vi "nodeInfo.get_process_info.vi"(5 "error in (no error)":errorcluster) -> (14 "numberProcs":i32, 15 "procNames":string[](array[string]), 16 "procID":i32[](array[numeric]), 17 "procMemory":i32[](array[numeric]), 18 "procRuntime":dbl[](array[numeric]), 19 "error out":errorcluster)   [LabVIEW 2014, in "LVNodeInfo.lvlib"]
doc: "Gets information about local processes."
uses:
  LVNodeInfo.lvlib
  <vilib>/Utility/error.llb/whitespace.ctl
  NodeMon/bin/libNodeInfo.dll
  NodeMon/bin/libNodeInfo.so
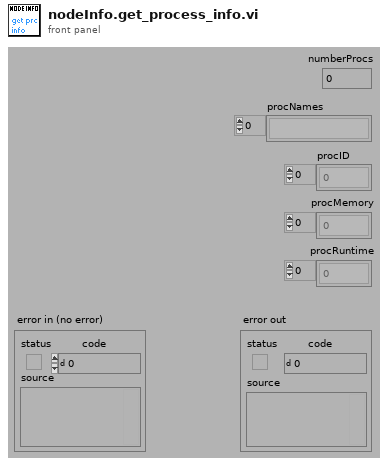
[diagram p1: front panel]
types:
  T1 = typedef "whitespace.ctl" = u16
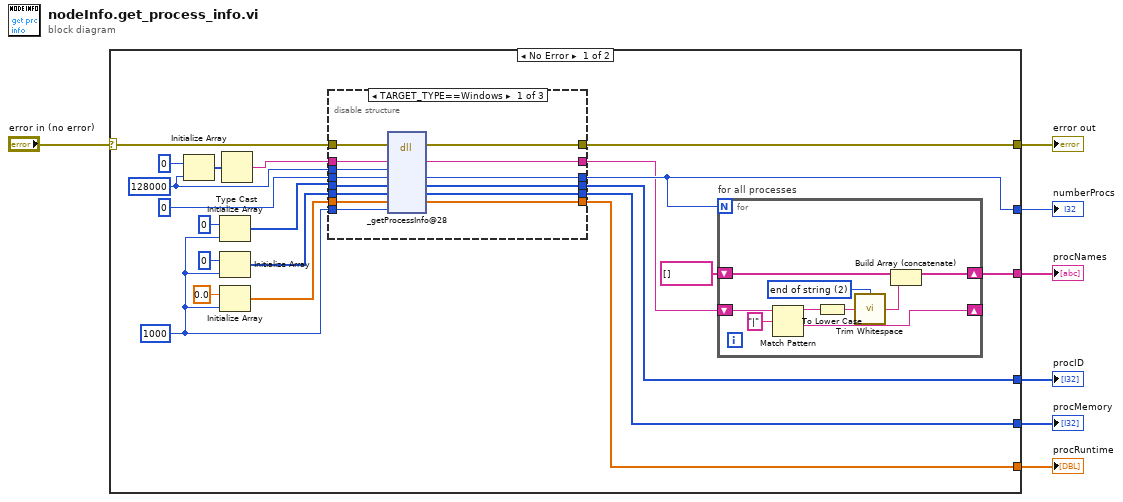
[diagram p0: block diagram]
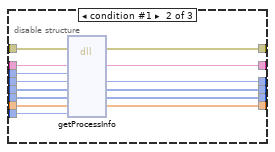
[diagram p2: hidden frame]
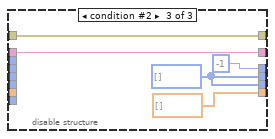
[diagram p3: hidden frame]
diagram:
  n1 = case shown="No Error" "error in (no error)" {
    selector: "error in (no error)" -> [w22 w71]
    tunnel: [w23 w71] -> w6
    tunnel: [w25 _] -> w5
    tunnel: [w24 _] -> w1
    tunnel: [w28 _] -> w4
    tunnel: [w27 _] -> w3
    tunnel: [w26 _] -> w2
    frame No Error {
      w12 = 1000 ("dimension size")
      w17 = 128000 ("dimension size")
      n2 = Initialize Array(i8 0, w17) -> (w20:i8[])
      n3 = Initialize Array(0 ("element"), w12) -> (w15:i32[])
      n4 = Initialize Array(0 ("element"), w12) -> (w11:i32[])
      n5 = Initialize Array(0.0 ("element"), w12) -> (w10:dbl[])
      n6 = Type Cast(x=w20) -> (*(type *) &x=w19:string)  [unwired: 1 in]
      n7 = disable-structure "Conditional Disable Structure" shown="TARGET_TYPE==Windows" {
        disable-tunnel: [w42 w56 w58] -> w28
        disable-tunnel: [w41 w55 w58] -> w27
        disable-tunnel: [w40 w54 dbl[] [] ("procRuntime")] -> w26
        disable-tunnel: [w39 w53 -1 ("numberProcs")] -> w25
        disable-tunnel: w19 -> [w38 w52 w60]
        disable-tunnel: 0 ("numberProcs") -> [w37 w51 _]
        disable-tunnel: w17 -> [w36 w50 _]
        disable-tunnel: w15 -> [w35 w49 _]
        disable-tunnel: w12 -> [w34 w48 _]
        disable-tunnel: w11 -> [w33 w47 _]
        disable-tunnel: w10 -> [w32 w46 _]
        disable-tunnel: [w31 w45 w60] -> w9
        disable-tunnel: w22 -> [w30 w44 w61]
        disable-tunnel: [w29 w43 w61] -> w23
        frame condition #0 (active) {
          n8 = dll-call lib="D:/CS-Source/LV2014/GPL/lib.lib/DimLVEvent/NodeMon/bin/libNodeInfo.dll" fn="_getProcessInfo@28"(error in=w30, "procNames"=w38, "procNamesLen"=w36, "numberProcs"=w37, "procID"=w35, "procMemory"=w33, "procRuntime"=w32, "arraySize"=w34) -> (error out=w29:errorcluster, "procNames"=w31:string, "numberProcs"=w39:i32, "procID"=w42:i32[], "procMemory"=w41:i32[], "procRuntime"=w40:dbl[])  [unwired: 5 in, 1 out]
        }
        frame condition #1 {
          n9 = dll-call lib="D:/Git/CS-framework/CSlibraries/DimLVEvent/NodeMon/bin/libNodeInfo.so" fn="getProcessInfo" label="libNodeInfo.dll:_getProcessInfo@28"(error in=w44, "procNames"=w52, "procNamesLen"=w50, "numberProcs"=w51, "procID"=w49, "procMemory"=w47, "procRuntime"=w46, "arraySize"=w48) -> (error out=w43:errorcluster, "procNames"=w45:string, "numberProcs"=w53:i32, "procID"=w56:i32[], "procMemory"=w55:i32[], "procRuntime"=w54:dbl[])  [unwired: 5 in, 1 out]
        }
        frame condition #2 {
          w58 = i32[] [] ("procID")
        }
      }
      n10 = for "for all processes" {
        N: w25 -> [_]
        shift-right: [w65] -> w24
        shift-left: string[] [] -> [w67]
        shift-right: [w68] -> _
        shift-left: w9 -> [w70]
        w62 = T1 2 items=["both", "start of string", "end of string"] ("location (both)")
        n11 = Match Pattern(string=w70, regular expression="|") -> (before substring=w66:string, after substring=w68:string)  [unwired: 1 in, 2 out]
        n12 = To Lower Case(string=w66) -> (all lower case string=w64:string)
        n13 = call <vilib>:"Trim Whitespace.vi"("string"=w64, "location (both)"=w62) -> ("trimmed string"=w63:string)
        n14 = Build Array (concatenate)(w67, w63) -> (w65:string[])
      }
    }
    frame Error {
    }
  }
  "error out" <- w6
  "numberProcs" <- w5
  "procID" <- w4
  "procMemory" <- w3
  "procRuntime" <- w2
  "procNames" <- w1
